vi "Nav_CheckMinDistanceToNode.vi"(9 "Array of path nodes":T1, 11 "Robot current position":T2) -> (3 "Coordinates":T1)   [LabVIEW 2009, in "Navigation.lvlib"]
uses:
  Navigation.lvlib
  Nav_CordinateArray.ctl
  Drive/Drive_Utils.lvlib
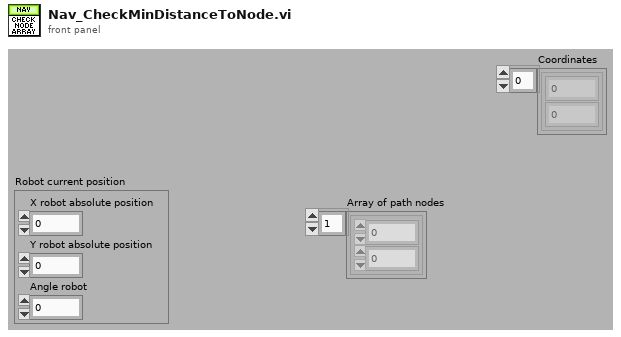
[diagram p1: front panel]
types:
  T1 = typedef "Navigation.lvlib/Nav_CordinateArray.ctl" = cluster{"X position":dbl, "Y position":dbl}[]
  T2 = cluster{"X robot absolute position":dbl, "Y robot absolute position":dbl, "Angle robot":dbl}
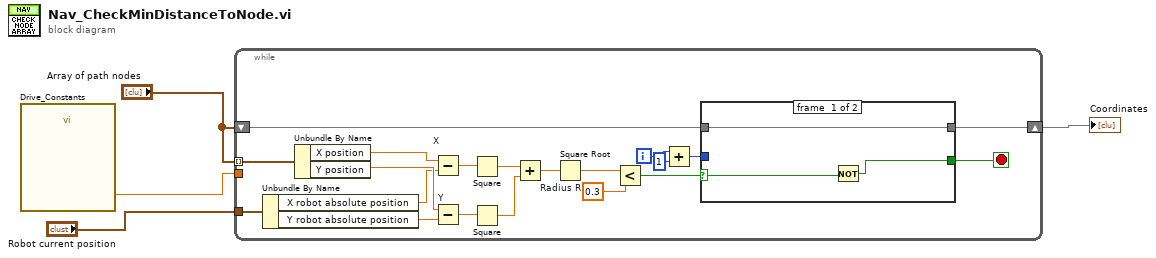
[diagram p0: block diagram]
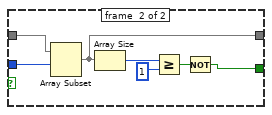
[diagram p2: hidden frame]
diagram:
  n1 = call "Drive_Constants.vi"() -> ("Position accuracy (m)"=w2:dbl)  [unwired: 19 in, 8 out]
  n2 = while {
    tunnel: "Array of path nodes" -> [w23] mode=indexing
    shift-right: [w10] -> w1
    shift-left: "Array of path nodes" -> [w11]
    tunnel: "Robot current position" -> [w24]
    tunnel: w2 -> [_]
    i -> [w7]
    stop <- w9 stop-if-true
    n3 = Unbundle By Name(w24) -> ("X robot absolute position"=w14:dbl, "Y robot absolute position"=w17:dbl)
    n4 = Unbundle By Name(w23) -> ("X position"=w15:dbl, "Y position"=w16:dbl)
    n5 = Subtract "X"(x=w15, y=w14) -> (x-y=w19:dbl)
    n6 = Subtract "Y"(x=w16, y=w17) -> (x-y=w18:dbl)
    n7 = Square(x=w19) -> (x^2=w22:dbl)
    n8 = Square(x=w18) -> (x^2=w20:dbl)
    n9 = Add(x=w22, y=w20) -> (x+y=w21:dbl)
    n10 = Square Root "Radius R"(x=w21) -> (sqrt(x)=w13:dbl)
    n11 = Less?(x=w13, y=0.3) -> (x < y?=w12:bool)
    n12 = Add(x=w7, y=1) -> (x+y=w8:i32)
    n13 = case shown="True" w12 {
      selector: w12 -> [w27 _]
      tunnel: w11 -> [w25 w34]
      tunnel: [w25 w30] -> w10
      tunnel: w8 -> [_ w33]
      tunnel: [w26 w28] -> w9
      frame #0 {
        n14 = Not(x=w27) -> (.not. x?=w26:bool)
      }
      frame #1 {
        n15 = Array Subset(array=w34, index=w33) -> (w30:T1)  [unwired: 1 in]
        n16 = Array Size(array=w30) -> (size(s)=w31:i32)
        n17 = Greater Or Equal?(x=w31, y=1) -> (x >= y?=w29:bool)
        n18 = Not(x=w29) -> (.not. x?=w28:bool)
      }
    }
  }
  "Coordinates" <- w1
